vi "cblas dsymv.vi"(0 "A":T3, 1 "x":dbl[](array[numeric]), 2 "y":dbl[](array[numeric]), 3 "alpha":dbl=1.0, 4 "beta":dbl=1.0, 5 "order":T2=101 items=["CblasRowMajor"=101, "CblasColMajor"=102], 7 "uplo":T1=121 items=["CblasUpper"=121, "CblasLower"=122], 8 "lda":i32, 10 "incx":i32=1, 11 "n":i32=-1, 12 "incy":i32=1) -> (14 "dsymv":dbl[](array[numeric]), 19 "error":i32)   [LabVIEW 2020, in "NI_AALBLAS.lvlib"]
uses:
  NI_AALBLAS.lvlib
  RealMatrix.ctl
  Order.ctl
  UpLo.ctl
  <resource>/lvblas.dll
  NI_Matrix.lvlib
panel:
  # "void cblas_dsymv(order, uplo, n, alpha, *A, lda, *x, incx, beta, *y, incy)"
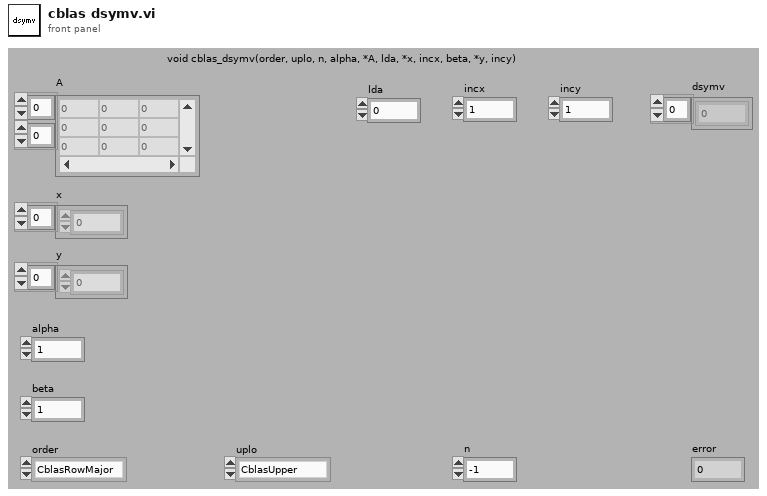
[diagram p1: front panel]
types:
  T1 = typedef "NI_AALBLAS.lvlib/UpLo.ctl" = i32
  T2 = typedef "NI_AALBLAS.lvlib/Order.ctl" = i32
  T3 = typedef "NI_Matrix.lvlib/RealMatrix.ctl" = dbl[][]
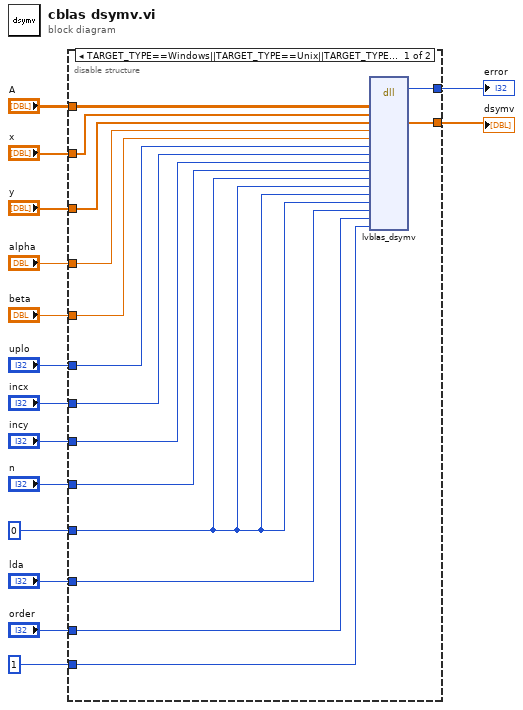
[diagram p0: block diagram]
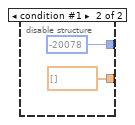
[diagram p2: hidden frame]
diagram:
  n1 = disable-structure shown="TARGET_TYPE==Windows||TARGET_TYPE==Unix||TARGET_TYPE==Mac||TARGET_TYPE==RT" {
    disable-tunnel: "x" -> [w30 _]
    disable-tunnel: "y" -> [w29 _]
    disable-tunnel: "alpha" -> [w28 _]
    disable-tunnel: [w27 dbl[] [] ("y")] -> w12
    disable-tunnel: "beta" -> [w26 _]
    disable-tunnel: "A" -> [w25 _]
    disable-tunnel: [w24 -20078 ("error")] -> w9
    disable-tunnel: 0 -> [w21 _]
    disable-tunnel: "lda" -> [w20 _]
    disable-tunnel: "uplo" -> [w23 _]
    disable-tunnel: "n" -> [w22 _]
    disable-tunnel: "order" -> [w19 _]
    disable-tunnel: "incx" -> [w18 _]
    disable-tunnel: "incy" -> [w17 _]
    disable-tunnel: 1 -> [w16 _]
    frame condition #0 (active) {
      n2 = dll-call lib="C:/Program Files (x86)/National Instruments/LabVIEW 2020/resource/lvblas.*" fn="lvblas_dsymv" ("CBLAS.dll:MtrxxVectH")("a"=w25, "x"=w30, "y"=w29, "alpha"=w28, "beta"=w26, "uplo"=w23, "IncX"=w18, "IncY"=w17, "n"=w22, "startARow"=w21, "startACol"=w21, "startX"=w21, "startY"=w21, "lda"=w20, "order"=w19, "check"=w16) -> ("error"=w24:i32, "y"=w27:dbl[])  [unwired: 18 in, 2 out]
    }
    frame condition #1 {
    }
  }
  "dsymv" <- w12
  "error" <- w9
